vi "sces-to-cmd-str-final.vi"(11 "模式列表":T2(array[cluster]) {"sce-pannel-list"."pannel"."ID" format="%02x"}) -> (3 "数组 3":cluster{"字符串":string, "数组 2":string[]}[](array[cluster]))   [LabVIEW 2019]
panel:
  out "sce-pannel-list out":T1(array[cluster]) {"pannel"."ID" format="%02x"}
  in  "模式列表 2":T2(array[cluster]) {"sce-pannel-list"."pannel"."ID" format="%02x"}
  in  "模式列表 3":T2(array[cluster])=[{"模式"="关|睡眠模式", "sce-pannel-list"=[{"pannel"=[{"ID"=1, "type"="dev", "flag"="", "name"="第三方", "Act"={"Attribute"="", "Action"="open", "Value"=0.0}}, {"ID"=2, "type"="dev", "flag"="", "name"="水电费", "Act"={"Attribute"="", "Action"="close", "Value"=0.0}}, {"ID"=3, "type"="dev", "flag"="", "name"="二", "Act"={"Attribute"="", "Action"="open", "Value"=0.0}}], "pannel-id"=1.0}, {"pannel"=[{"ID"=1, "type"="dev", "flag"="", "name"="而风蛋糕", "Act"={"Attribute"="", "Action"="open", "Value"=0.0}}, {"ID"=2, "type"="dev", "flag"="", "name"="官方", "Act"={"Attribute"="", "Action"="open", "Value"=0.0}}, {"ID"=3, "type"="dev", "flag"="", "name"="俄文", "Act"={"Attribute"="", "Action"="close", "Value"=0.0}}], "pannel-id"=2.0}]}, {"模式"="开|睡眠模式", "sce-pannel-list"=[{"pannel"=[{"ID"=1, "type"="dev", "flag"="", "name"="而风蛋糕", "Act"={"Attribute"="", "Action"="open", "Value"=0.0}}, {"ID"=2, "type"="dev", "flag"="", "name"="官方", "Act"={"Attribute"="", "Action"="open", "Value"=0.0}}, {"ID"=3, "type"="dev", "flag"="", "name"="俄文", "Act"={"Attribute"="", "Action"="close", "Value"=0.0}}], "pannel-id"=2.0}]}, {"模式"="起床模式", "sce-pannel-list"=[{"pannel"=[{"ID"=1, "type"="dev", "flag"="", "name"="而风蛋糕", "Act"={"Attribute"="", "Action"="open", "Value"=0.0}}, {"ID"=2, "type"="dev", "flag"="", "name"="官方", "Act"={"Attribute"="", "Action"="open", "Value"=0.0}}, {"ID"=3, "type"="dev", "flag"="", "name"="俄文", "Act"={"Attribute"="", "Action"="close", "Value"=0.0}}], "pannel-id"=2.0}]}] {"sce-pannel-list"."pannel"."ID" format="%02x"}
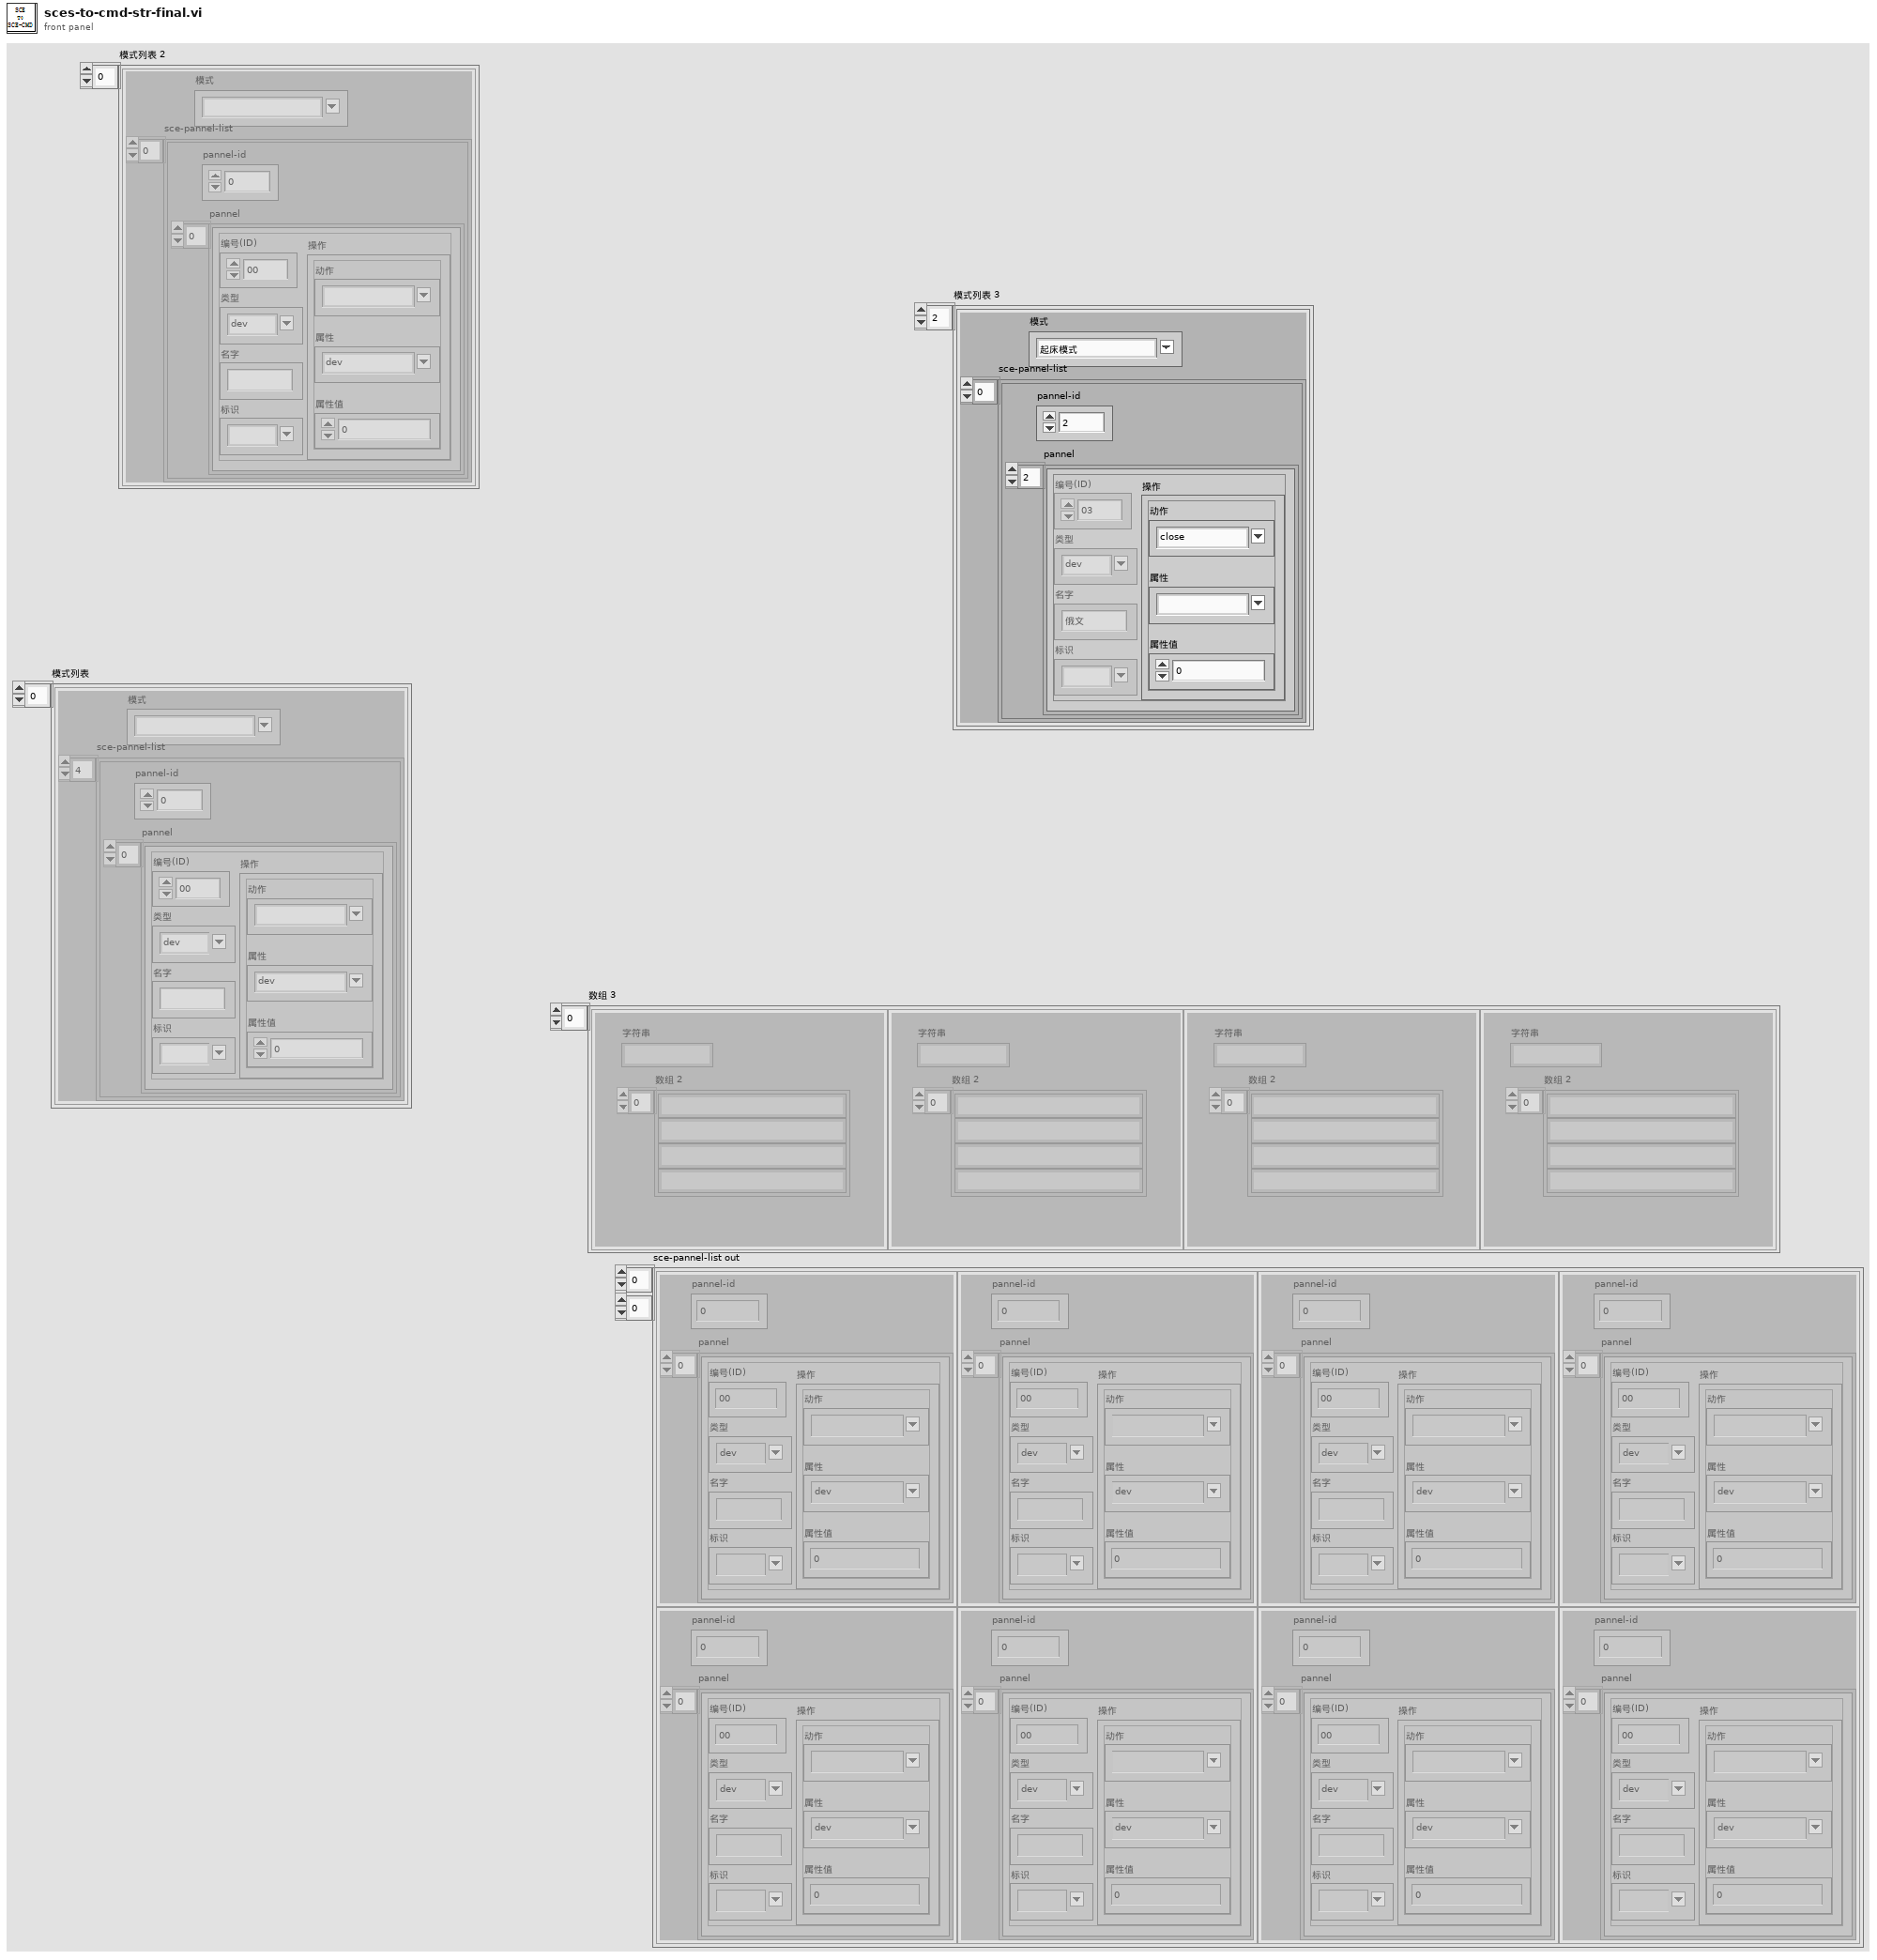
[diagram p1: front panel]
types:
  T1 = cluster{"pannel":cluster{"ID":u8, "type":string, "flag":string, "name":string, "Act":cluster{"Attribute":string, "Action":string, "Value":dbl}}[], "pannel-id":dbl}[][]
  T2 = cluster{"模式":string, "sce-pannel-list":cluster{"pannel":cluster{"ID":u8, "type":string, "flag":string, "name":string, "Act":cluster{"Attribute":string, "Action":string, "Value":dbl}}[], "pannel-id":dbl}[]}[]
  T3 = cluster{"pannel":cluster{"ID":u8, "type":string, "flag":string, "name":string, "Act":cluster{"Attribute":string, "Action":string, "Value":dbl}}[], "pannel-id":dbl}[]
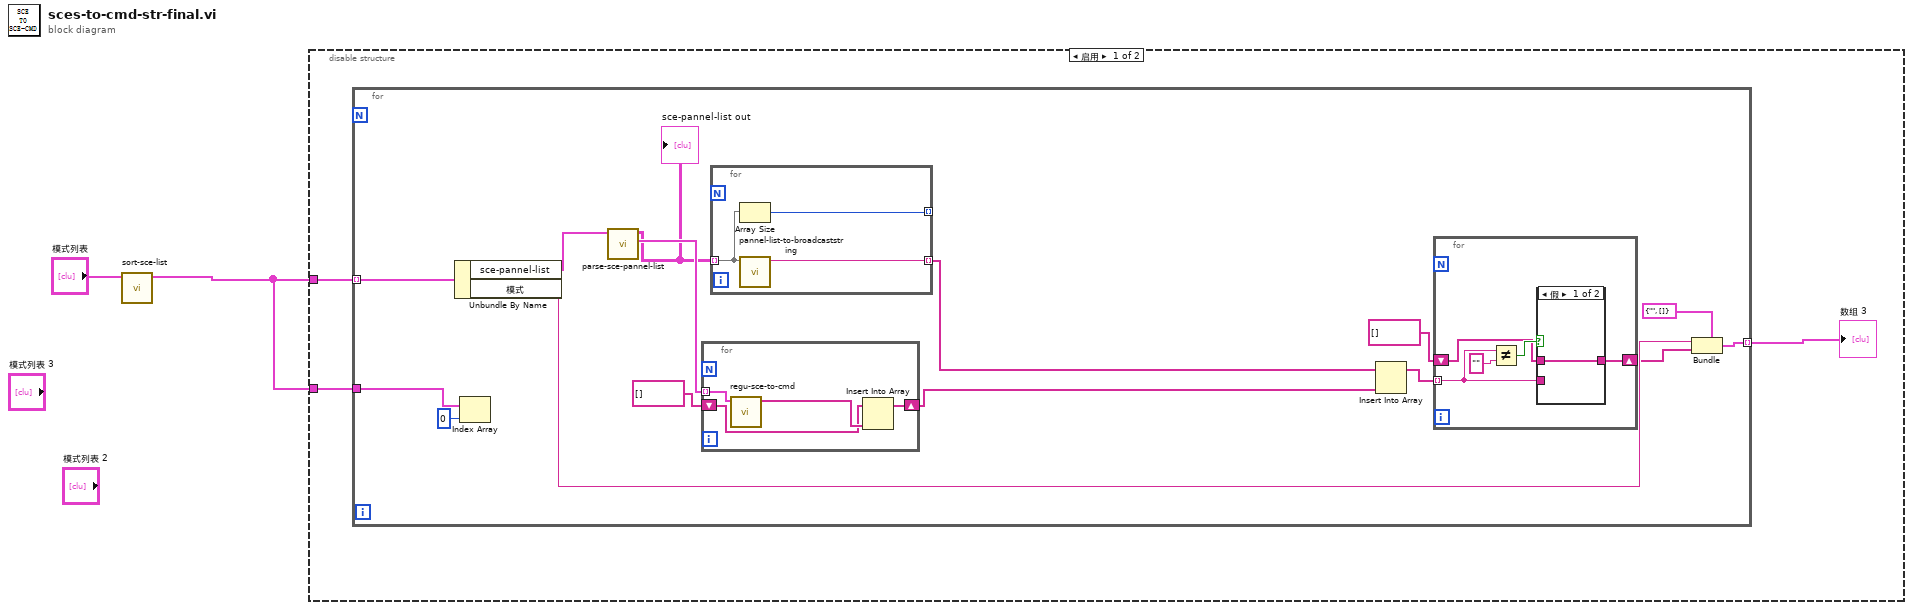
[diagram p0: block diagram]
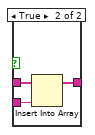
[diagram p2: hidden frame]
diagram:
  n1 = call "sort-sce-list.vi"("模式列表"="模式列表") -> ("模式列表-sorted"=w2:T2)  [unwired: 10 in]
  n2 = disable-structure shown="启用" {
    disable-tunnel: w2 -> [w5 _]
    disable-tunnel: w2 -> [w3 _]
    frame Enabled {
      n3 = for {
        tunnel: w5 -> [w6] mode=indexing
        tunnel: [w17] -> w4 mode=indexing
        tunnel: w3 -> [w12]
        n4 = Unbundle By Name(w6) -> ("sce-pannel-list"=w20:T3, "模式"=w18:string)
        n5 = Index Array(array=w12, index=0 ("索引")) -> ()  [unwired: 1 out]
        n6 = call "parse-sce-pannel-list.vi"("sce-pannel-list"=w20) -> ("sce-regulate-list"=w13:T3, "sce-pannel-list out"=w7:T1)  [unwired: 9 in]
        "sce-pannel-list out" <- w7
        n7 = for {
          tunnel: w13 -> [w24] mode=indexing
          shift-right: [w22] -> w8
          shift-left: string[] [] -> [w21]
          n8 = call "regu-sce-to-cmd.vi"("regulate-pannel"=w24) -> ("regulate-cmd"=w23:string[])  [unwired: 10 in]
          n9 = Insert Into Array(array=w21, new element=w23) -> (w22:string[])  [unwired: 1 in]
        }
        n10 = for {
          tunnel: w7 -> [w26] mode=indexing
          tunnel: [w27] -> w9 mode=indexing
          tunnel: [w25] -> _ mode=indexing
          n11 = Array Size(array=w26) -> (size(s)=w25:i32)
          n12 = call "pannel-list-to-broadcaststring.vi"("sce-pannel-list"=w26) -> ("sce-pannel-list-cmd"=w27:string)  [unwired: 10 in]
        }
        n13 = Insert Into Array(array=w9, new element=w8) -> (w15:string[])  [unwired: 1 in]
        n14 = for {
          tunnel: w15 -> [w30] mode=indexing
          shift-right: [w29] -> w14
          shift-left: string[] [] -> [w28]
          n15 = Not Equal?(x=w30, y="") -> (x != y?=w31:bool)
          n16 = case shown="假" w31 {
            tunnel: w30 -> [_ w36]
            tunnel: [w33 w35] -> w29
            tunnel: w28 -> [w33 w34]
            frame False {
            }
            frame True {
              n17 = Insert Into Array(array=w34, new element=w36) -> (w35:string[])  [unwired: 1 in]
            }
          }
        }
        n18 = Bundle(cluster=cluster{"字符串":string, "数组 2":string[]} {"字符串"="", "数组 2"=[]} ("簇"), "字符串"=w18, "数组 2"=w14) -> (w17:cluster{"字符串":string, "数组 2":string[]})
      }
      "数组 3" <- w4
    }
    frame Disabled {
    }
  }
